vi "Read queue reference.vi"(8 "error in (no error)":errorcluster) -> (0 "error out":errorcluster, 3 "ALA_Display_Queue ref":refnum<queue>)   [LabVIEW 2020, in "queue_display_loop_1.lvlib"]
uses:
  queue_display_loop_1.lvlib
  PTRL/dev_and_debug_tools/QueueMessage typedef.ctl
  library_variable.vi
  PTRL/dev_and_debug_tools/dev_and_debug_tools.lvlib
panel:
  # "Development\ncontrols/indicators useful for development and testing, but which are not outputs of the VI"
  # "Input\nInputs to the VI"
  # "Output\nOutputs of the VI"
  # "Description\n\nBlank VI with error handling case. \n\nSummarize the use of this VI in this space."
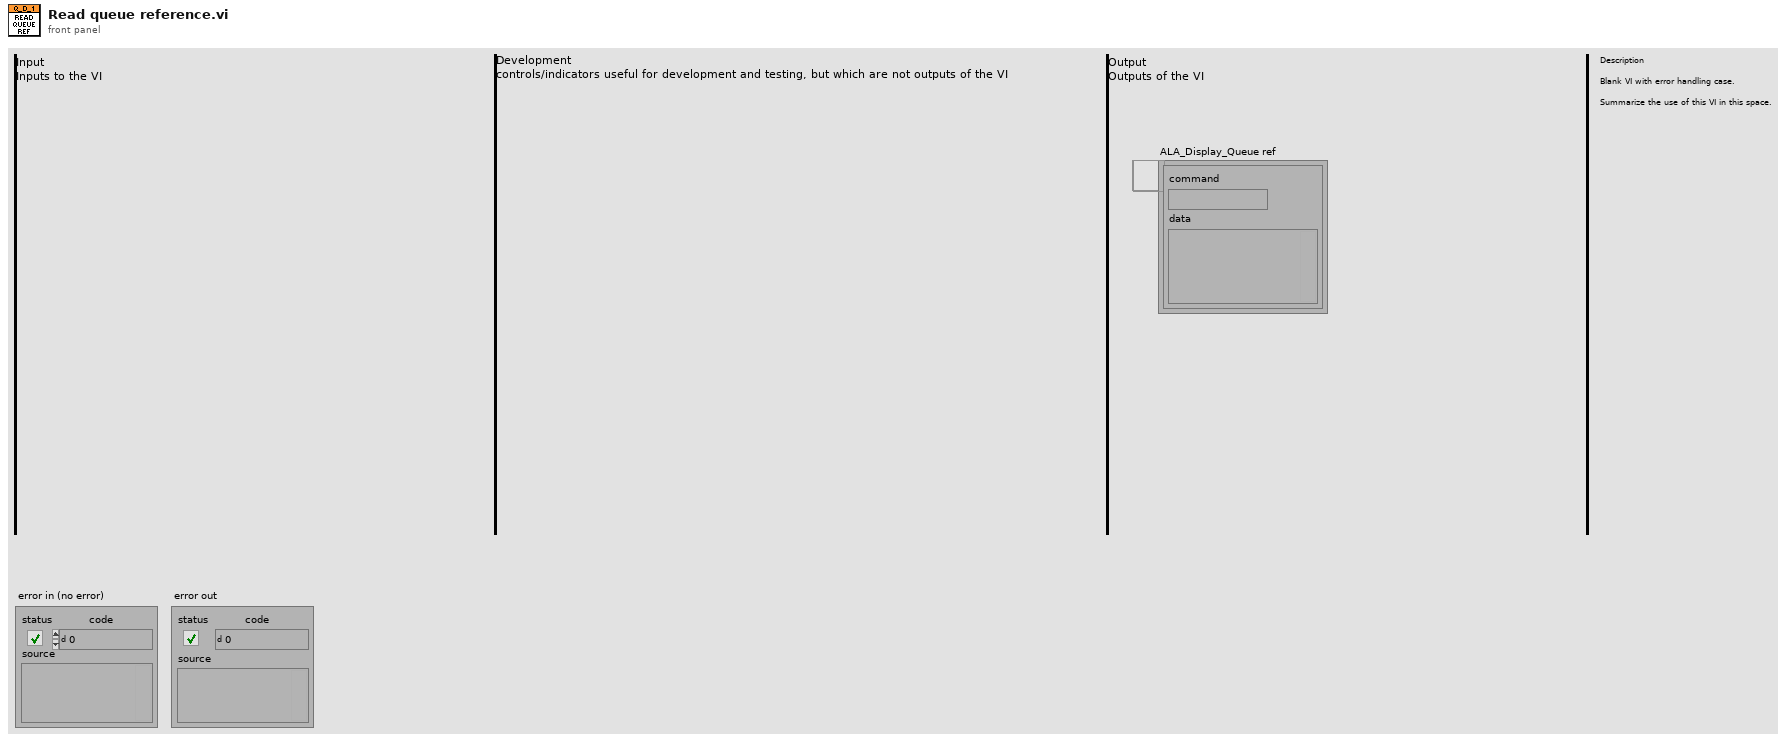
[diagram p1: front panel]
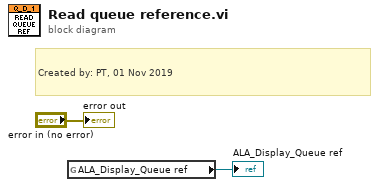
[diagram p0: block diagram]
diagram:
  # "Created by: PT, 01 Nov 2019"
  n1 = global read "library_variable.vi" "ALA_Display_Queue ref"() -> (→"ALA_Display_Queue ref":refnum<queue>)
  "error out" <- "error in (no error)"
